vi "Boulder Intake Control Controller.vi"(8 "error in":errorcluster) -> ()   [LabVIEW 2015]
doc: "This VI executes continuously carrying out the current operation and responding to updates or new operations. It will often contain the timing or control code that is difficult to place directly in TeleOp. This VI generally opens all sensors and motors and isolates the rest of the robot code from knowing how the operations are carried out."
uses:
  Boulder Intake Control Setpoints.ctl
  Boulder Intake Control Operations.ctl
  <vilib>/Rock Robotics/Network Tables/NT Write Boolean.vi
panel:
  out "Current\nCmd":string
  # "Tip: It may be helpful to observe inputs and sensor values.\nYou may also want to display tuning or debugging controls."
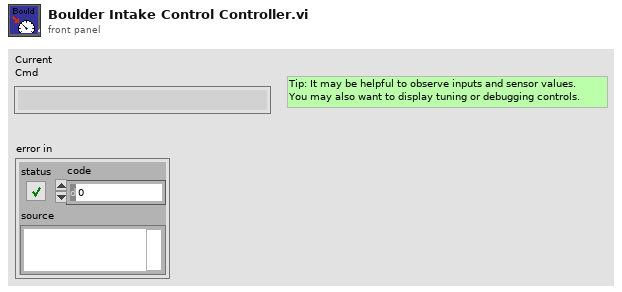
[diagram p1: front panel]
types:
  T1 = typedef "Boulder Intake Control Setpoints.ctl" = cluster{"Operation":T2, "Setpoint":dbl, "Duration":dbl}
  T2 = typedef "Boulder Intake Control Operations.ctl" = enum16{"Reserve", "Read Current", "Immediate", "Pickup", "Dump"}
  T3 = typedef "Command Status Info.ctl" = cluster{"Name":string, "Status":T4, "notifier out":T5}
  T4 = typedef "Completion Status.ctl" = enum16{"Successful", "Aborted", "Incomplete"}
  T5 = typedef "Completion Notifier.ctl" = refnum<notifier>
  T6 = cluster{"Default Command":T1, "Command Timing":cluster{"Start Time (ms)":u32, "Iterations":i32}, "Command Arguments":cluster{"Command Info":T3, "Description":string, "Default Command":T1, "notifier out":refnum<notifier>, "Subsystem Name":string}}
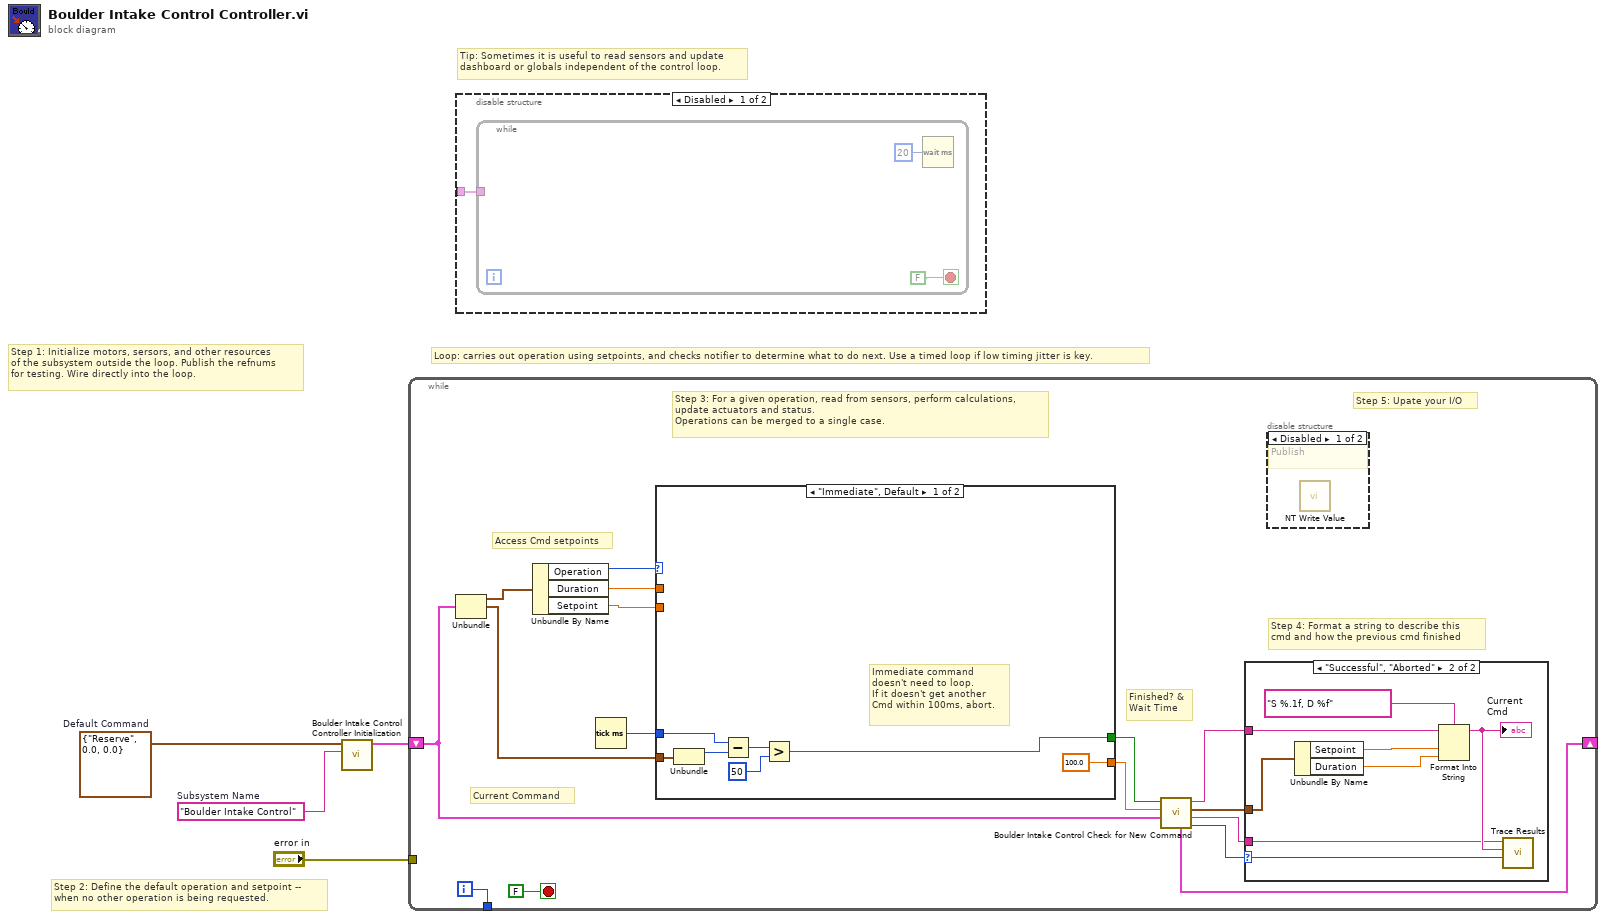
[diagram p0: block diagram]
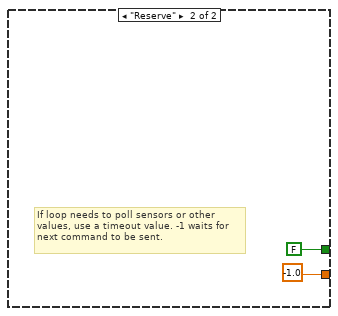
[diagram p5: hidden frame]
diagram:
  w1 = T1 {"Operation"=enum."Reserve", "Setpoint"=0.0, "Duration"=0.0}  # Default Command
  w2 = "Boulder Intake Control"  # Subsystem Name
  # "Tip: Sometimes it is useful to read sensors and update\ndashboard or globals independent of the control loop."
  # "Step 2: Define the default operation and setpoint --\nwhen no other operation is being requested."
  # "Step 1: Initialize motors, sersors, and other resources\nof the subsystem outside the loop. Publish the refnums\nfor testing. Wire directly into the loop."
  # "Loop: carries out operation using setpoints, and checks notifier to determine what to do next. Use a timed loop if low timing jitter is key."
  n1 = call "Boulder Intake Control Controller Initialization.vi"("Subsystem Name"=w2, "Default Command"=w1) -> ("Command Info"=w3:T6)  [unwired: 9 in]
  n2 = while {
    shift-right: [w11] -> _
    shift-left: w3 -> [w12]
    tunnel: [w19] -> _
    tunnel: "error in" -> [_]
    i -> [w19]
    stop <- FALSE stop-if-true
    # "Step 5: Upate your I/O"
    # "Step 4: Format a string to describe this\ncmd and how the previous cmd finished"
    # "Current Command"
    # "Access Cmd setpoints"
    # "Finished? &\nWait Time"
    # "Step 3: For a given operation, read from sensors, perform calculations,\nupdate actuators and status.\nOperations can be merged to a single case."
    n3 = Unbundle(w12) -> ("Default Command"=w18:T1, "Command Timing"=w14:cluster{"Start Time (ms)":u32, "Iterations":i32})  [unwired: 1 out]
    n4 = Unbundle By Name(w18) -> ("Operation"=w17:T2, "Duration"=w16:dbl, "Setpoint"=w13:dbl)
    n5 = Tick Count (ms)() -> (millisecond timer value=w15:u32)
    n6 = case shown="\"Immediate\", Default" w17 {
      tunnel: [100.0 -1.0] -> w9
      tunnel: [w29 FALSE ("ignore previous (F)")] -> w10
      tunnel: w14 -> [w31 _]
      tunnel: w16 -> [_ _]
      tunnel: w15 -> [w30 _]
      tunnel: w13 -> [_ _]
      frame "Immediate", Default {
        # "Immediate command\ndoesn't need to loop.\nIf it doesn't get another\nCmd within 100ms, abort."
        n7 = Unbundle(w31) -> ("Start Time (ms)"=w34:u32)  [unwired: 1 out]
        n8 = Subtract(x=w30, y=w34) -> (x-y=w33:u32)
        n9 = Greater?(x=w33, y=u8 50 ("Left Motor")) -> (0:w29:bool)
      }
      frame "Reserve" {
        # "If loop needs to poll sensors or other\nvalues, use a timeout value. -1 waits for\nnext command to be sent."
      }
    }
    n10 = call "Boulder Intake Control Check for New Command.vi"("Current Command"=w12, "Wait time (ms)"=w9, "Finished?"=w10) -> ("Completion"=w5:T4, "Subsystem Name"=w6:string, "Current Command"=w7:T1, "Initial Trace String"=w8:string, "NextCommand"=w11:T6)  [unwired: 4 in]
    n11 = case shown="\"Successful\", \"Aborted\"" w5 {
      selector: w5 -> [_ w28]
      tunnel: w8 -> [_ w24]
      tunnel: w7 -> [_ w25]
      tunnel: w6 -> [_ w21]
      frame "Incomplete", Default {
        # "Continuing current command"
      }
      frame "Successful", "Aborted" {
        # "Report and setup for next command"
        n12 = Unbundle By Name(w25) -> ("Setpoint"=w27:dbl, "Duration"=w22:dbl)
        n13 = Format Into String(format string="S %.1f, D %f", initial string=w24, w27, w22) -> (resulting string=w23:string)  [unwired: 1 in, 1 out]
        "Current\nCmd" <- w23
        n14 = call <vilib>:"Trace Results.vi"("Status of previous command"=w28, "Description"=w23, "Subsystem"=w21) -> ()  [unwired: 9 in]
      }
    }
    n15 = disable-structure shown="Disabled" {
      frame Disabled {
        # "Publish"
        n16 = call-poly <vilib>:"NT Write Value.vi"() -> ()  [unwired: 11 in, 1 out]
      }
      frame Enabled {
      }
    }
  }
  n17 = disable-structure shown="Disabled" {
    disable-tunnel: _ -> [w38 _]
    frame Disabled {
      n18 = while {
        tunnel: w38 -> [_]
        stop <- FALSE stop-if-true
        n19 = Wait (ms)(milliseconds to wait=u32 20) -> ()  [unwired: 1 out]
      }
    }
    frame Enabled {
    }
  }
